vi "Get Version.vi"(8 "error in (no error)":errorcluster, 11 "UDP Configurations in":refnum<class "UDP Configurations.lvclass">) -> (0 "error out":errorcluster, 2 "version":T1, 3 "UDP Configurations out":refnum<class "UDP Configurations.lvclass">)   [LabVIEW 2017, in "UDP Transceiver.lvlib" / "UDP Configurations.lvclass"]
uses:
  UDP Configurations.lvclass
  DSF Core.lvlibp/Typedefs/DSF Version Info.ctl
  DSF Core.lvlibp
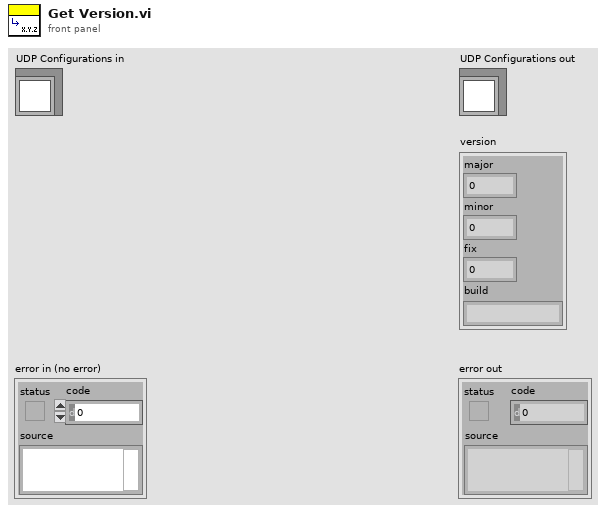
[diagram p1: front panel]
types:
  T1 = typedef "DSF Core.lvlibp/DSF Version Info.ctl" = cluster{"major":u32, "minor":u32, "fix":u32, "build":string}
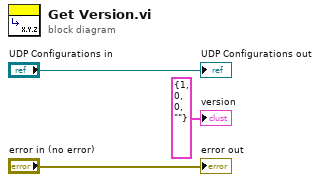
[diagram p0: block diagram]
diagram:
  "error out" <- "error in (no error)"
  "UDP Configurations out" <- "UDP Configurations in"
  "version" <- T1 {"major"=1, "minor"=0, "fix"=0, "build"=""} ("version")
